vi "hidSPD Close Multi Sessions.vi"(8 "error in (no error)":errorcluster, 11 "spdDevSessions out":T1[](array[typedef]) {"hidSPD.Controller"."HV_bias" format="%#_6p, V"; "hidSPD.Controller"."TSet" format="%#_6p, DegC"}) -> (0 "error out":errorcluster)   [LabVIEW 2018, in "hidSPDLibForLabView.lvlib"]
uses:
  hidSPDLibForLabView.lvlib
  hidSPD Controls/hidSPD Device Session.ctl
  hidSPD Controls/hidSPD Controller.ctl
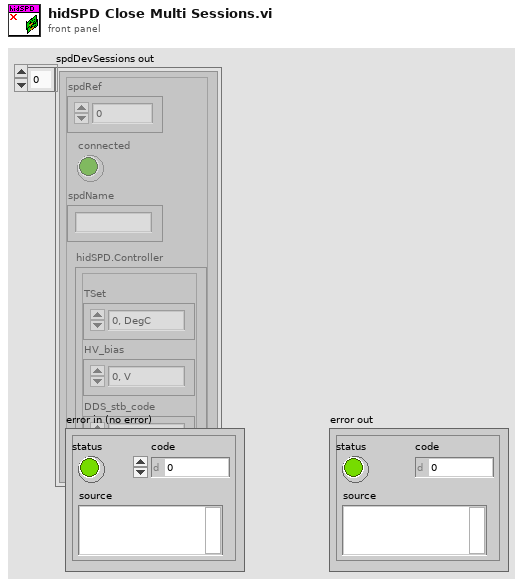
[diagram p1: front panel]
types:
  T1 = typedef "hidSPDLibForLabView.lvlib/hidSPD Device Session.ctl" = cluster{"spdRef":u64, "connected":bool, "spdName":string, "hidSPD.Controller":T2}
  T2 = typedef "hidSPDLibForLabView.lvlib/hidSPD Controller.ctl" = cluster{"TSet":sgl, "HV_bias":sgl, "DDS_stb_code":u16}
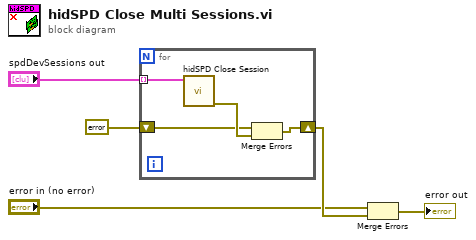
[diagram p0: block diagram]
diagram:
  n1 = for {
    tunnel: "spdDevSessions out" -> [w9] mode=indexing
    shift-right: [w8] -> w3
    shift-left: errorcluster {"status"=FALSE, "code"=0, "source"=""} ("error in (no error)") -> [w6]
    n2 = call "hidSPD Close Session.vi"("spdDevHandle"=w9) -> ("error out"=w7:errorcluster)  [unwired: 10 in]
    n3 = Merge Errors(w6, w7) -> (w8:errorcluster)
  }
  n4 = Merge Errors("error in (no error)", w3) -> (→"error out":errorcluster)
